vi "Validate.vi"(8 "error in":errorcluster, 10 "parameters":variant, 11 "CEF_HierarchyRepo in":refnum<class "CEF_HierarchyRepo.lvclass">) -> (0 "error out":errorcluster, 3 "CEF_HierarchyRepo out":refnum<class "CEF_HierarchyRepo.lvclass">)   [LabVIEW 2023, in "CEF.lvlib" / "CEF_HierarchyRepo.lvclass"]
doc: "Copyright 2017 National Instruments Corporation\n\nLicensed under the Apache License, Version 2.0 (the \"License\"); you may not use this file except in compliance with the License. You may obtain a copy of the License at http://www.apache.org/licenses/LICENSE-2.0\nUnless required by applicable law or agreed to in writing, software distributed under the License is distributed on an \"AS IS\" BASIS, WITHOUT WARRANTIES OR CONDITIONS OF ANY KIND, either express or implied. See the License for the specific language governing permissions and limitations under the License."
uses:
  CEF_HierarchyRepo.lvclass
  CEF_HierarchyRepo.lvclass/CEF_HierarchyRepo.ctl
  serializable configuration/CEF_serializable configuration.lvclass
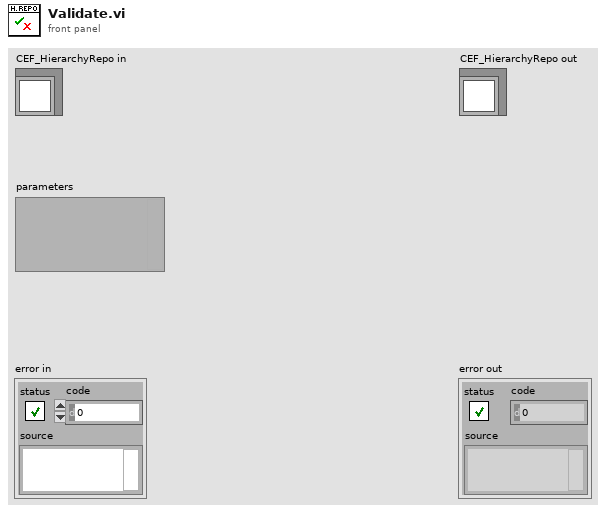
[diagram p1: front panel]
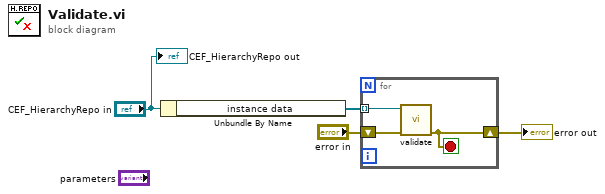
[diagram p0: block diagram]
diagram:
  n1 = Unbundle By Name("CEF_HierarchyRepo in") -> ("instance data"=w1:refnum<class "CEF_serializable configuration.lvclass">[])
  n2 = for {
    shift-right: [w6] -> w2
    shift-left: "error in" -> [w7]
    tunnel: w1 -> [w5] mode=indexing
    stop <- w6 stop-if-true
    n3 = call-dynamic "validate.vi"("error in"=w7, "CEF_Configuration in"=w5) -> ("error out"=w6:errorcluster)  [unwired: 8 in, 1 out]
  }
  "error out" <- w2
  "CEF_HierarchyRepo out" <- "CEF_HierarchyRepo in"
